vi "List Slots.vi"(5 "Password":string, 7 "User Name":string, 8 "error in (no error)":errorcluster, 11 "serverName In":string) -> (0 "error out":errorcluster, 1 "Resources out":refnum<k20>[](array[refnum]), 2 "Session out":refnum<k21>, 3 "Refnum out":refnum<k20>, 4 "NumSlots":i32)   [LabVIEW 2019, in "SEECD System Explorer.lvlib"]
doc: "List slots (supporting property \"Slot Programming Mode\") populated.\nThis VI also returns number of chassis slots (typically 4 or 8)."
uses:
  <vilib>/nisyscfg/Filter Mode.ctl
  <vilib>/nisyscfg/Close (Resources).vi
  SEECD System Explorer.lvlib
  <vilib>/nisyscfg/nisyscfg.lvlib
  <resource>/objmgr/nisysapi.rc
  <resource>/objmgr/nicontrollersysapi.rc
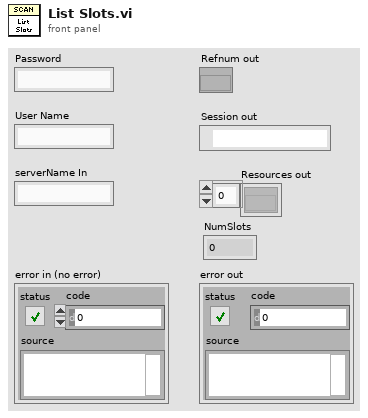
[diagram p1: front panel]
types:
  T1 = typedef "nisyscfg.lvlib/Filter Mode.ctl" = i32
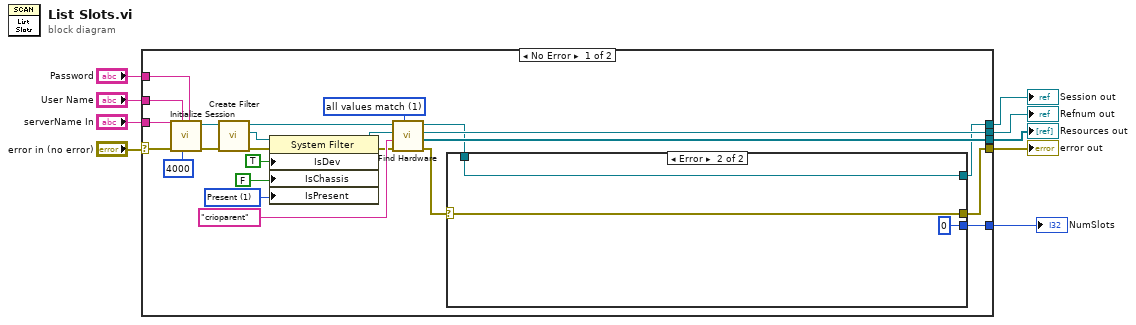
[diagram p0: block diagram]
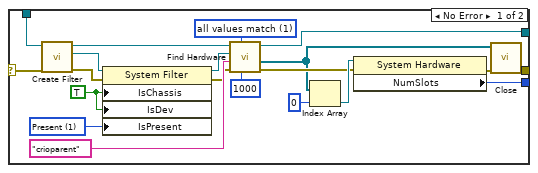
[diagram p2: hidden frame]
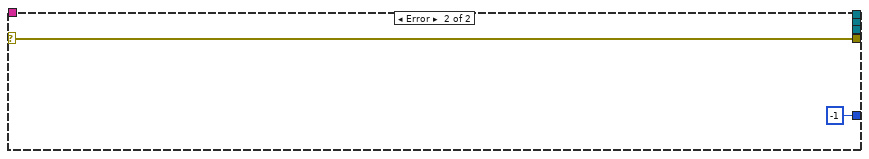
[diagram p3: hidden frame]
diagram:
  n1 = case shown="No Error" "error in (no error)" {
    selector: "error in (no error)" -> [w17 w58]
    tunnel: [w33 _] -> w9
    tunnel: [w12 w58] -> w8
    tunnel: [w13 _] -> w7
    tunnel: [w21 _] -> w6
    tunnel: "Password" -> [w20 _]
    tunnel: "User Name" -> [w19 _]
    tunnel: "serverName In" -> [w18 _]
    tunnel: [w11 -1 ("NumSlots")] -> w1
    frame No Error {
      w31 = 1 items=["Initializing"=-2, "Unknown"=-1, "Not Present"=0, "Present"=1] ("Devices & Chassis:Is Present")
      w27 = T1 1 items=["all values match"=1, "any value matches"=2, "values do not match"=3, "all properties exist"=4] ("filter mode (all values match)")
      n2 = call <vilib>:"Initialize Session.vi"("Password"=w20, "Connect Timeout (4000 ms)"=u32 4000, "User Name"=w19, "error in (no error)"=w17, "Target (localhost)"=w18) -> ("error out"=w16:errorcluster, "Session out"=w15:refnum<k21>)  [unwired: 5 in]
      n3 = call <vilib>:"Create Filter.vi"("error in (no error)"=w16, "Session in"=w15) -> ("error out"=w22:errorcluster, "Filter out"=w23:refnum<k20>, "Session out"=w24:refnum<k21>)  [unwired: 7 in]
      n4 = property class="System Filter"(reference=w23, error in=w22, "IsDev"=TRUE ("Is Device"), "IsChassis"=FALSE ("Is Chassis"), "IsPresent"=w31) -> (reference out=w26:refnum<k20>, error out=w25:errorcluster)
      n5 = call <vilib>:"Find Hardware.vi"("Filter Mode (all values match)"=w27, "error in (no error)"=w25, "Experts"="crioparent" ("Expert Info:Expert Name"), "Filter in"=w26, "Session in"=w24) -> ("error out"=w10:errorcluster, "Resources out"=w21:refnum<k20>[], "Filter out"=w33:refnum<k20>, "Session out"=w14:refnum<k21>)  [unwired: 3 out]
      n6 = case shown="Error" w10 {
        selector: w10 -> [w41 w56]
        tunnel: w14 -> [w50 w55]
        tunnel: [w49 w55] -> w13
        tunnel: [w44 w56] -> w12
        tunnel: [w42 0 ("NumSlots")] -> w11
        frame No Error {
          w52 = T1 1 items=["all values match"=1, "any value matches"=2, "values do not match"=3, "all properties exist"=4] ("filter mode (all values match)")
          w35 = 1 items=["Initializing"=-2, "Unknown"=-1, "Not Present"=0, "Present"=1] ("Devices & Chassis:Is Present")
          w36 = TRUE ("Is Chassis")
          n7 = call <vilib>:"Create Filter.vi"("error in (no error)"=w41, "Session in"=w50) -> ("error out"=w37:errorcluster, "Filter out"=w40:refnum<k20>, "Session out"=w53:refnum<k21>)  [unwired: 7 in]
          n8 = property class="System Filter"(reference=w40, error in=w37, "IsChassis"=w36, "IsDev"=w36, "IsPresent"=w35) -> (reference out=w39:refnum<k20>, error out=w38:errorcluster)
          n9 = call <vilib>:"Find Hardware.vi"("Remote Timeout (300,000 ms)"=u32 1000, "Filter Mode (all values match)"=w52, "error in (no error)"=w38, "Experts"="crioparent", "Filter in"=w39, "Session in"=w53) -> ("error out"=w46:errorcluster, "Resources out"=w43:refnum<k20>[], "Session out"=w49:refnum<k21>)  [unwired: 3 out]
          n10 = Index Array(array=w43, index=0) -> (element=w47:refnum<k20>)
          n11 = property class="System Hardware"(reference=w47, error in=w46) -> (error out=w45:errorcluster, "NumSlots"=w42:i32)  [unwired: 1 out]
          n12 = call-poly <vilib>:"Close.vi"("error in (no error)"=w45, "Resources in"=w43) -> ("error out"=w44:errorcluster)  [unwired: 9 in]
        }
        frame Error {
        }
      }
    }
    frame Error {
    }
  }
  "Refnum out" <- w9
  "error out" <- w8
  "Session out" <- w7
  "Resources out" <- w6
  "NumSlots" <- w1
